vi "RMS to Pk-Pk.vi"(1 "RMS":dbl=1.0 format="%.3f") -> (0 "pk-pk":dbl=nan format="%.3f")   [LabVIEW 2010]
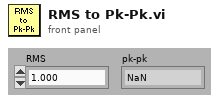
[diagram p1: front panel]
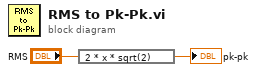
[diagram p0: block diagram]
diagram:
  n1 = expression code="2 * x * sqrt(2)"("RMS") -> (→"pk-pk":dbl)
